vi "Prueba_Entorno.vi"(1 "Posición":cluster{"X":dbl, "Y":dbl, "Z":dbl}, 2 "Mundo":path=path "C:/Users/LuisFernando/Documents/UPIITA/8vo semestre/Instrumentacion Virtual Aplicada/Solidworks/Sistema_Coordenado/Archivos Blender/Mundo/Mundo.wrl", 3 "Objetos_Moviles":path=path "C:/Users/LuisFernando/Documents/UPIITA/8vo semestre/Instrumentacion Virtual Aplicada/Solidworks/Sistema_Coordenado/Archivos Blender/Archivos_moviles", 4 "Objetos_Constantes":path=path "C:/Users/LuisFernando/Documents/UPIITA/8vo semestre/Instrumentacion Virtual Aplicada/Solidworks/Sistema_Coordenado/Archivos Blender/Archivos_constantes") -> (0 "3D Picture":refnum<vi>(3d-picture))   [LabVIEW 2017]
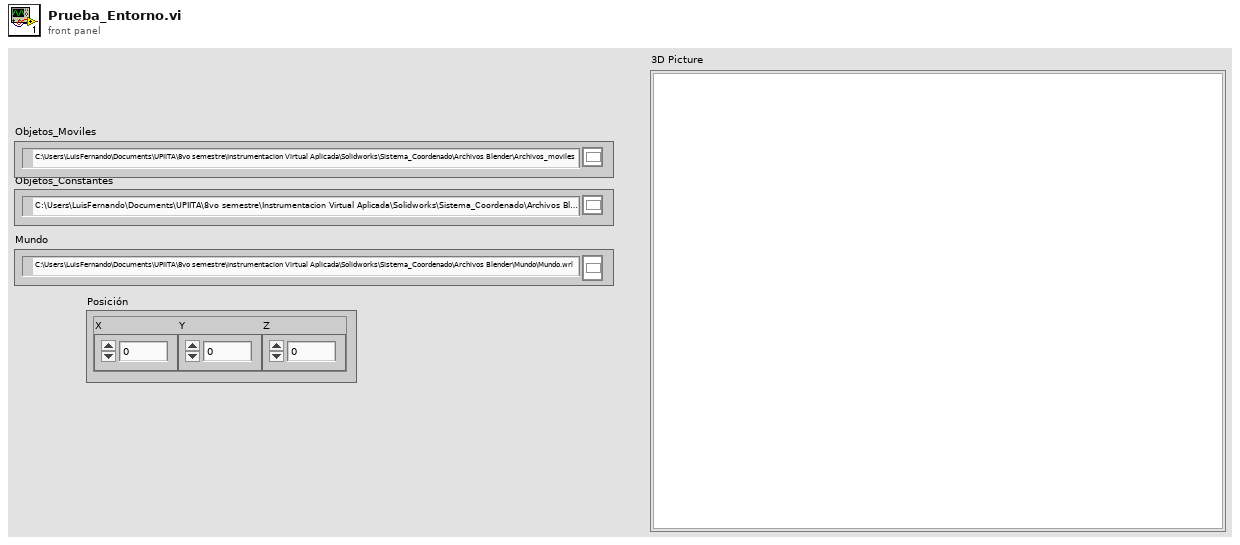
[diagram p1: front panel]
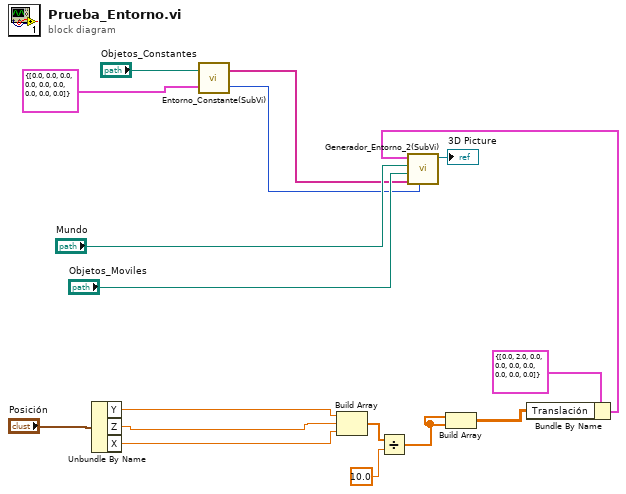
[diagram p0: block diagram]
diagram:
  n1 = Unbundle By Name("Posición") -> ("Y"=w3:dbl, "Z"=w2:dbl, "X"=w1:dbl)
  n2 = call "Entorno_Constante(SubVi).vi"("Cluster"=cluster{"Translación":dbl[][]} {"Translación"=[[0.0, 0.0, 0.0], [0.0, 0.0, 0.0], [0.0, 0.0, 0.0]]} ("Cluster_Constante"), "Objetos"="Objetos_Constantes") -> ("Archivos"=w4:i32, "Salida_Texto"=w13:string[])
  n3 = Build Array(w3, w2, w1) -> (w7:dbl[])
  n4 = Divide(x=w7, y=10.0) -> (x/y=w6:dbl[])
  n5 = Build Array(w6, w6) -> (w9:dbl[][])
  n6 = Bundle By Name(cluster=cluster{"Translación":dbl[][]} {"Translación"=[[0.0, 2.0, 0.0], [0.0, 0.0, 0.0], [0.0, 0.0, 0.0]]} ("Cluster"), "Translación"=w9) -> (w8:cluster{"Translación":dbl[][]})
  n7 = call "Generador_Entorno_2(SubVi).vi"("Archivos_Constantes"=w4, "Entrada de Texto"=w13, "Objetos"="Objetos_Moviles", "Mundo"="Mundo", "Cluster"=w8) -> ("3D Picture"=→"3D Picture":refnum<vi>)  [unwired: 6 in]
